vi "RecordExist.vi"(11 "Machine":string) -> ()   [LabVIEW 2012]
uses:
  <vilib>/addons/database/NI_Database_API.lvlib
  <vilib>/addons/database/Connection.llb/DB Tools Open Connec (Path).vi
panel:
  in  "Cust_lot":string
  out "date/time string":string
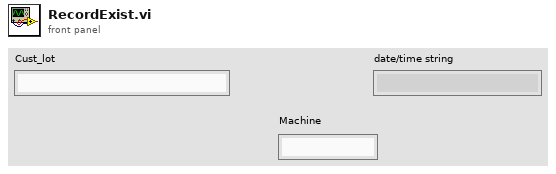
[diagram p1: front panel]
types:
  T1 = typedef "NI_Database_API.lvlib/Conn ObjectReference.ctl" = refnum<k1>
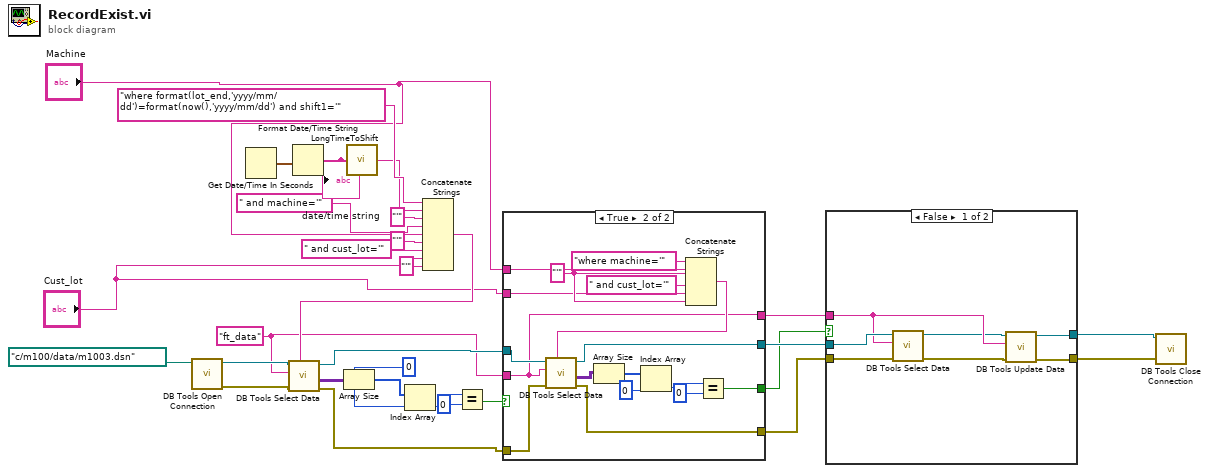
[diagram p0: block diagram]
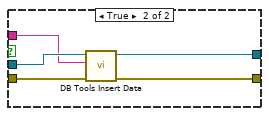
[diagram p2: hidden frame]
diagram:
  w9 = "ft_data" ("table")
  n1 = call-poly <vilib>:"DB Tools Open Connection.vi"("connection information"=path "c:/m100/data/m1003.dsn") -> ("error out"=w19:errorcluster, "connection reference"=w20:T1)  [unwired: 7 in]
  n2 = Get Date/Time In Seconds() -> (seconds since 1Jan1904=w29:timestamp)
  n3 = Format Date/Time String(seconds (now)=w29) -> (date/time string=w28:string)  [unwired: 2 in]
  "date/time string" <- w28
  n4 = call "LongTimeToShift.vi"("input string"=w28) -> ("s? t:f"=w26:string)  [unwired: 1 in]
  n5 = Concatenate Strings("where format(lot_end,'yyyy/mm/dd')=format(now(),'yyyy/mm/dd') and shift1='" ("condition"), w26, "'" ("string"), " and machine='", "Machine", "'" ("string"), " and cust_lot='" ("string"), "Cust_lot", "'" ("string")) -> (w10:string)
  n6 = call <vilib>:"DB Tools Select Data.vi"("condition"=w10, "error in (no error)"=w19, "table"=w9, "connection reference"=w20) -> ("error out"=w11:errorcluster, "data"=w16:variant[][], "connection reference out"=w12:T1)  [unwired: 2 in]
  n7 = Array Size(array=w16) -> (size(s)=w18:i32[])
  n8 = Index Array(array=w18, index=0) -> (element=w15:i32)
  n9 = Equal?(x=w15, y=0) -> (x = y?=w13:bool)
  n10 = case shown="True" w13 {
    tunnel: w12 -> [w32 w50]
    tunnel: w11 -> [w31 w49]
    tunnel: w9 -> [w33 w34]
    tunnel: "Machine" -> [_ w45]
    tunnel: "Cust_lot" -> [_ w44]
    tunnel: [_ w37] -> w4
    tunnel: [w32 w36] -> w6
    tunnel: [w31 w35] -> w5
    tunnel: [w33 w34] -> w1
    frame False {
    }
    frame True {
      w48 = "'" ("string")
      n11 = Concatenate Strings("where machine='" ("string"), w45, w48, " and cust_lot='" ("string"), w44, w48) -> (w43:string)
      n12 = call <vilib>:"DB Tools Select Data.vi"("condition"=w43, "error in (no error)"=w49, "table"=w34, "connection reference"=w50) -> ("error out"=w35:errorcluster, "data"=w42:variant[][], "connection reference out"=w36:T1)  [unwired: 2 in]
      n13 = Array Size(array=w42) -> (size(s)=w41:i32[])
      n14 = Index Array(array=w41, index=0) -> (element=w39:i32)
      n15 = Equal?(x=w39, y=0) -> (x = y?=w37:bool)
    }
  }
  n16 = case shown="False" w4 {
    tunnel: w6 -> [w55 w62]
    tunnel: w5 -> [w54 w61]
    tunnel: [w57 w60] -> w3
    tunnel: [w56 w59] -> w2
    tunnel: w1 -> [w53 w58]
    frame False {
      n17 = call <vilib>:"DB Tools Select Data.vi"("error in (no error)"=w54, "table"=w53, "connection reference"=w55) -> ("error out"=w51:errorcluster, "connection reference out"=w52:T1)  [unwired: 3 in, 1 out]
      n18 = call <vilib>:"DB Tools Update Data.vi"("error in (no error)"=w51, "table"=w53, "connection reference"=w52) -> ("error out"=w56:errorcluster, "connection reference out"=w57:T1)  [unwired: 7 in]
    }
    frame True {
      n19 = call <vilib>:"DB Tools Insert Data.vi"("error in (no error)"=w61, "table"=w58, "connection reference"=w62) -> ("error out"=w59:errorcluster, "connection reference out"=w60:T1)  [unwired: 7 in]
    }
  }
  n20 = call <vilib>:"DB Tools Close Connection.vi"("error in (no error)"=w2, "connection reference"=w3) -> ()  [unwired: 5 in, 1 out]
